vi "comled.vi"(1 "Dato_ACK":u8) -> (0 "Led_ACK":T1)   [LabVIEW 2019]
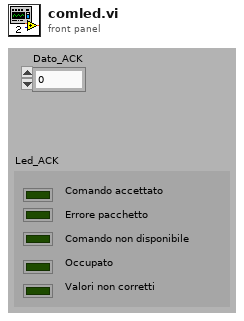
[diagram p1: front panel]
types:
  T1 = cluster{"Comando accettato":bool, "Errore pacchetto":bool, "Comando non disponibile":bool, "Occupato":bool, "Valori non corretti":bool}
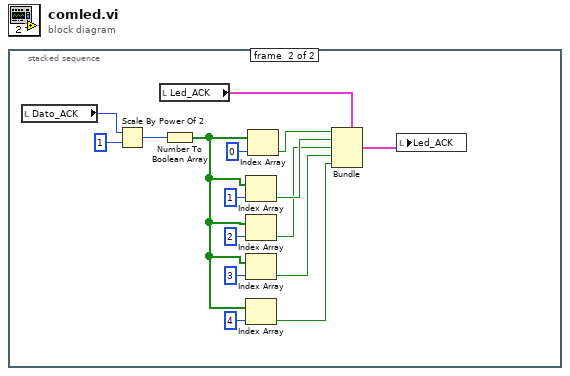
[diagram p0: block diagram]
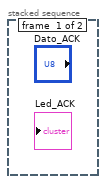
[diagram p2: hidden frame]
diagram:
  n1 = stacked-sequence {
    frame #0 {
    }
    frame #1 {
      n2 = local read "Dato_ACK"() -> (w15:u8)
      n3 = Scale By Power Of 2(n=w15, x=u8 1) -> (x*2^n=w14:u8)
      n4 = local read "Led_ACK"() -> (w13:T1)
      n5 = Number To Boolean Array(number=w14) -> (Boolean array=w3:bool[])
      n6 = Index Array(array=w3, index=1) -> (element=w7:bool)
      n7 = Index Array(array=w3, index=2) -> (element=w6:bool)
      n8 = Index Array(array=w3, index=3) -> (element=w5:bool)
      n9 = Index Array(array=w3, index=4) -> (element=w1:bool)
      n10 = Index Array(array=w3, index=0) -> (element=w8:bool)
      n11 = Bundle(cluster=w13, "Comando accettato"=w8, "Errore pacchetto"=w7, "Comando non disponibile"=w6, "Occupato"=w5, "Valori non corretti"=w1) -> (w4:T1)
      n12 = local write "Led_ACK"(w4) -> ()
    }
  }
